vi "Test Better MessageBox.vi"   [LabVIEW 2015]
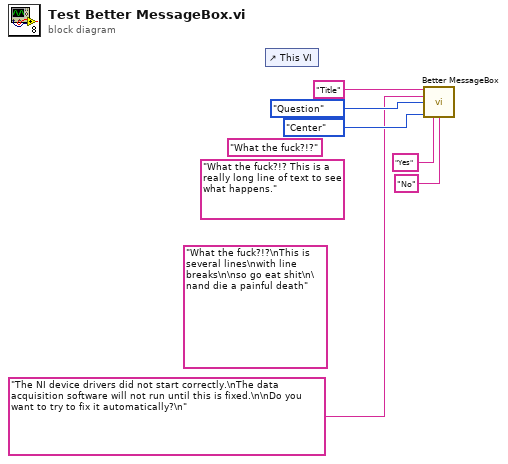
[diagram p0: block diagram]
diagram:
  (unwired) "What the fuck?!?\nThis is several lines\nwith line breaks\n\nso go eat shit\n\nand die a painful death" ("Message")
  (unwired) "What the fuck?!?"
  (unwired) "What the fuck?!? This is a really long line of text to see what happens." ("Message")
  n1 = control-ref of="This VI"() -> ()  [unwired: 1 out]
  n2 = call "Better MessageBox.vi"("Title"="Title", "Message"="The NI device drivers did not start correctly.\nThe data acquisition software will not run until this is fixed.\n\nDo you want to try to fix it automatically?\n", "Icon Style"=enum16{"Warning", "Error", "Info", "Question"}."Question", "Text.Justification"=enum16{"Left", "Center", "Right"}."Center", "Yes text"="Yes", "No text"="No") -> ()  [unwired: 9 in, 1 out]
